vi "cRIO Main.vi"() -> ()   [LabVIEW 2013]
doc: "This example runs a background service that initializes and interacts with the Tag Bus Data framework. The service is designed to run continuously so that the framework can be reinitialized with a new configuration without rebooting the target. This can save time when iterating on a configuration.\n\nThe example includes a collection of VIs for sending and receiving messages from the engine service."
uses:
  SubVIs/command commands to rtexe process.ctl
  SubVIs/engine status data.ctl
  <vilib>/NI/Module Execution Interface/Engine Runtime/Execution States.ctl
  <vilib>/NI/Module Execution Interface/Engine Runtime/Fault.ctl
  <vilib>/NI/Tag Bus Module Framework/runtime/error classification.ctl
  SubVIs/queue name.ctl
  <vilib>/NI/AMC/Read Termination Message.vi
  SubVIs/command to string.vi
  SubVIs/string to commands.vi
  <vilib>/NI/AMC/Create Single Message.vi
  <vilib>/NI/AMC/Globals.vi
  TBD execution service.lvlib
  <vilib>/NI/AMC/AMC.lvlib
  <vilib>/NI/Module Execution Interface/Engine Runtime/Engine Runtime Interface.lvclass
  <vilib>/NI/Tag Bus Module Framework/runtime/TBM module execution interface.lvclass
panel:
  in  "target alias":string="cRIO"
  in  "Exit":bool
  in  "Reload":bool
  out "final error":errorcluster
  out "system error":errorcluster
  out "engine statuses":T1[](array[typedef])
  out "command error":errorcluster
  out "recent command":T5
  out "engine loaded":string
  out "load error":errorcluster
  out "invalid message":string
  in  "config. file path":path=path "/home/lvuser/natinst/bin/FullSystem.pcfg"
  # "status information"
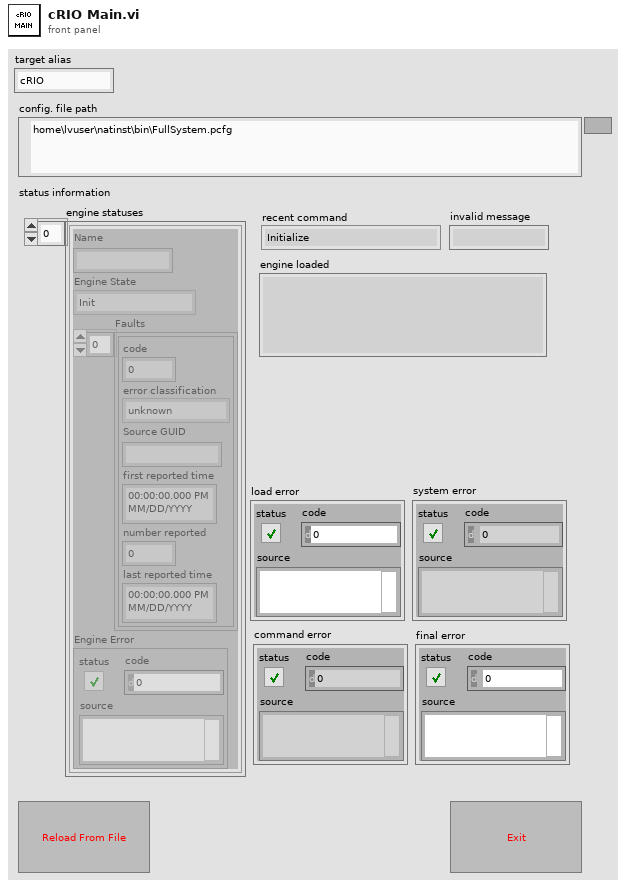
[diagram p1: front panel]
types:
  T1 = typedef "TBD execution service.lvlib/engine status data.ctl" = cluster{"Name":string, "Engine State":T2, "Faults":T3[], "Engine Error":errorcluster}
  T2 = typedef "Engine Runtime Interface.lvclass/Execution States.ctl" = enum16{"Init", "Pre-Operational", "Safe-Operational", "Operational", "Stopped"}
  T3 = typedef "Engine Runtime Interface.lvclass/Fault.ctl" = cluster{"code":i32, "error classification":T4, "Source GUID":string, "first reported time":timestamp, "number reported":u32, "last reported time":timestamp}
  T4 = typedef "TBM module execution interface.lvclass/error classification.ctl" = enum16{"unknown", "none", "trivial", "recoverable", "critical"}
  T5 = typedef "TBD execution service.lvlib/command commands to rtexe process.ctl" = enum16{"Initialize", "Add Search Paths", "Load from File", "Unload File", "Open All Engines", "Open Single Engine", "Initialize All Engines", "Initialize Single Engine", "Start All", "Start Single", "Pause All", "Pause Single", "Stop All", "Stop Single", "Close All", "Close Single", "Set Safe State All", "Set Safe State Single", "Get Status", "Exit", "Error", "Load Bitfile", "Unload Bitfile", "Clear Faults Single", "Clear Faults All"}
  T6 = typedef "TBD execution service.lvlib/queue name.ctl" = enum16{"TOrtmainexec", "FROMrtmainexec"}
  T7 = typedef "AMC.lvlib/Message Queue.ctl" = refnum<queue>
  T8 = typedef "TBD execution service.lvlib/common reponses to network process.ctl" = enum16{"System Error", "Load Report", "Action Response", "Engine Status"}
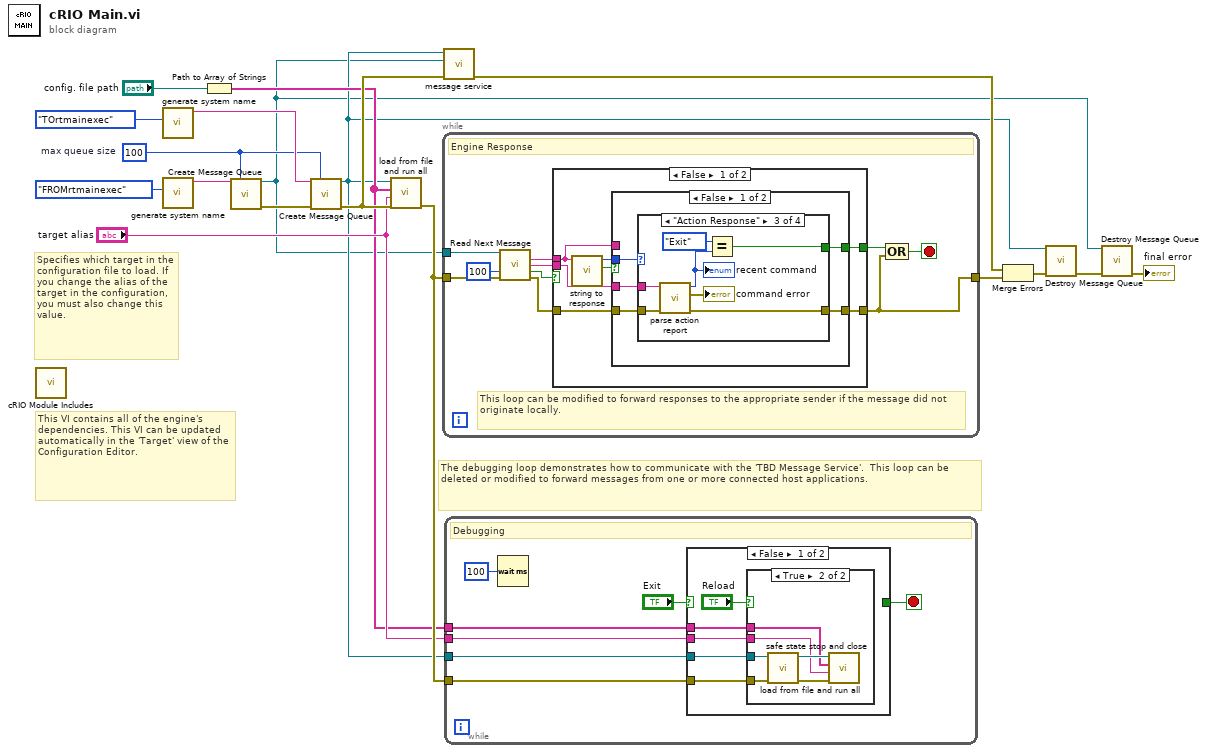
[diagram p0: block diagram]
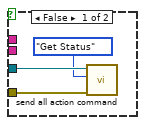
[diagram p2: hidden frame]
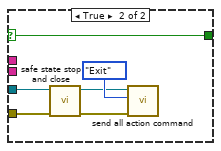
[diagram p3: hidden frame]
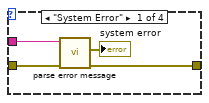
[diagram p4: hidden frame]
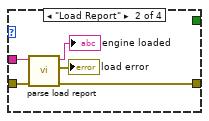
[diagram p5: hidden frame]
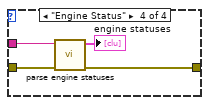
[diagram p6: hidden frame]
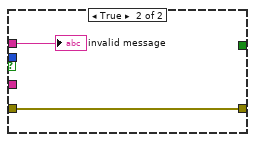
[diagram p7: hidden frame]
diagram:
  w12 = 100  # max queue size
  # "This VI contains all of the engine's dependencies. This VI can be updated automatically in the 'Target' view of the Configuration Editor."
  # "Specifies which target in the configuration file to load. If you change the alias of the target in the configuration, you must also change this value."
  # "The debugging loop demonstrates how to communicate with the 'TBD Message Service'.  This loop can be deleted or modified to forward messages from one or more connected host applications."
  n1 = call "cRIO Module Includes.vi"() -> ()  [unwired: 12 in]
  n2 = call "generate system name.vi"("queue type"=queue_name."TOrtmainexec" ("queue")) -> ("queue name"=w16:string)  [unwired: 10 in]
  n3 = call "generate system name.vi"("queue type"=queue_name."FROMrtmainexec" ("queue")) -> ("queue name"=w18:string)  [unwired: 10 in]
  n4 = Path to Array of Strings(0:"config. file path") -> (2:w8:string[])  [unwired: 1 out]
  n5 = call <vilib>:"Create Message Queue.vi"("message queue name"=w18, "max queue size (-1, unlimited)"=w12) -> ("message queue out"=w1:T7, "error out"=w17:errorcluster)  [unwired: 12 in]
  n6 = call <vilib>:"Create Message Queue.vi"("message queue name"=w16, "max queue size (-1, unlimited)"=w12, "error in"=w17) -> ("message queue out"=w2:T7, "error out"=w11:errorcluster)  [unwired: 11 in]
  n7 = call "load from file and run all.vi"("error in"=w11, "target alias"="target alias", "tokenized path"=w8, "message queue in"=w2) -> ("error out"=w10:errorcluster)  [unwired: 6 in, 1 out]
  n8 = while {
    tunnel: w1 -> [w27]
    tunnel: w10 -> [w24]
    tunnel: [w19] -> w7
    stop <- w21 stop-if-true
    # "This loop can be modified to forward responses to the appropriate sender if the message did not originate locally."
    # "Engine Response"
    n9 = call <vilib>:"Read Next Message.vi"("message queue in"=w27, "timeout (1 ms)"=100, "error in"=w24) -> ("message name"=w26:string, "message value"=w20:string, "timed out?"=w23:bool, "error out"=w25:errorcluster)  [unwired: 5 in, 4 out]
    n10 = case shown="False" w23 {
      tunnel: w26 -> [w29 _]
      tunnel: [w34 _] -> w22
      tunnel: w25 -> [w32 w63]
      tunnel: [w31 w63] -> w19
      tunnel: w20 -> [w30 _]
      frame False {
        n11 = call "string to response.vi"("command string"=w29) -> ("invalid"=w35:bool, "responses"=w33:T8)  [unwired: 9 in]
        n12 = case shown="False" w35 {
          tunnel: w30 -> [w39 _]
          tunnel: [w36 _] -> w34
          tunnel: w33 -> [w40 _]
          tunnel: w32 -> [w38 w62]
          tunnel: [w37 w62] -> w31
          tunnel: w29 -> [_ w61]
          frame False {
            n13 = case shown="\"Action Response\"" w40 {
              tunnel: w39 -> [w44 w49 w56 w60]
              tunnel: w38 -> [w43 w48 w55 w59]
              tunnel: [w41 w45 w53 w58] -> w37
              tunnel: [_ _ w50 _] -> w36
              frame "System Error" {
                n14 = call "parse error message.vi"("error in"=w43, "message data"=w44) -> ("error out"=w41:errorcluster, "system error"=→"system error":errorcluster)  [unwired: 8 in]
              }
              frame "Load Report" {
                n15 = call "parse load report.vi"("error in"=w48, "message data"=w49) -> ("error out"=w45:errorcluster, "load error"=→"load error":errorcluster, "engine loaded"=→"engine loaded":string)  [unwired: 7 in]
              }
              frame "Action Response" {
                n16 = call "parse action report.vi"("error in"=w55, "message data"=w56) -> ("error out"=w53:errorcluster, "command error"=→"command error":errorcluster, "commands"=w52:T5)  [unwired: 7 in]
                "recent command" <- w52
                n17 = Equal?(x=command_commands_to_rtexe_process."Exit", y=w52) -> (x = y?=w50:bool)
              }
              frame "Engine Status" {
                n18 = call "parse engine statuses.vi"("error in"=w59, "message data"=w60) -> ("error out"=w58:errorcluster, "engine statuses"=→"engine statuses":T1[])  [unwired: 8 in]
              }
            }
          }
          frame True {
            "invalid message" <- w61
          }
        }
      }
      frame True {
      }
    }
    n19 = Compound Arithmetic op=OR(w22, w19) -> (w21:bool)
  }
  n20 = call "message service.vi"("error in"=w11, "response queue"=w1, "command queue"=w2) -> ("error out"=w6:errorcluster)  [unwired: 8 in]
  n21 = while {
    tunnel: w10 -> [w68]
    tunnel: w2 -> [w69]
    tunnel: w8 -> [w67]
    tunnel: "target alias" -> [w66]
    stop <- w65 stop-if-true
    # "Debugging"
    n22 = Wait (ms)(milliseconds to wait=u32 100) -> ()  [unwired: 1 out]
    n23 = case shown="False" "Exit" {
      selector: "Exit" -> [_ w88]
      tunnel: w69 -> [w74 w90]
      tunnel: w68 -> [w73 w89]
      tunnel: w67 -> [w72 _]
      tunnel: w66 -> [w71 _]
      tunnel: [_ w88] -> w65
      frame False {
        n24 = case shown="True" "Reload" {
          tunnel: w74 -> [w78 w84]
          tunnel: w73 -> [w77 w83]
          tunnel: w72 -> [_ w80]
          tunnel: w71 -> [_ w79]
          frame False {
            n25 = call "send all action command.vi"("error in"=w77, "commands"=command_commands_to_rtexe_process."Get Status", "message queue in"=w78) -> ()  [unwired: 7 in, 2 out]
          }
          frame True {
            n26 = call "safe state stop and close.vi"("error in"=w83, "message queue in"=w84) -> ("error out"=w81:errorcluster, "message queue out"=w82:T7)  [unwired: 8 in]
            n27 = call "load from file and run all.vi"("error in"=w81, "target alias"=w79, "tokenized path"=w80, "message queue in"=w82) -> ()  [unwired: 6 in, 2 out]
          }
        }
      }
      frame True {
        n28 = call "safe state stop and close.vi"("error in"=w89, "message queue in"=w90) -> ("error out"=w85:errorcluster, "message queue out"=w86:T7)  [unwired: 8 in]
        n29 = call "send all action command.vi"("error in"=w85, "commands"=command_commands_to_rtexe_process."Exit", "message queue in"=w86) -> ()  [unwired: 7 in, 2 out]
      }
    }
  }
  n30 = Merge Errors(w6, w7) -> (w3:errorcluster)
  n31 = call <vilib>:"Destroy Message Queue.vi"("message queue in"=w2, "error in"=w3) -> ("error out"=w5:errorcluster)  [unwired: 11 in, 2 out]
  n32 = call <vilib>:"Destroy Message Queue.vi"("message queue in"=w1, "error in"=w5) -> ("error out"=→"final error":errorcluster)  [unwired: 11 in, 2 out]
